vi "Memory.Pointer.In Range.vi"(8 "error in (no error)":errorcluster, 9 "offset":u64 format="%d bytes", 10 "length":i64 format="%d bytes", 11 "Pointer in":refnum<class "Memory.Pointer.lvclass">) -> (0 "error out":errorcluster, 2 "in range?":bool, 3 "Pointer out":refnum<class "Memory.Pointer.lvclass">)   [LabVIEW 2016, in "LabVIEW Memory Manager.lvlib" / "Memory.Pointer.lvclass"]
uses:
  Memory.Pointer.lvclass
  Memory.Pointer.lvclass/Memory.Pointer.ctl
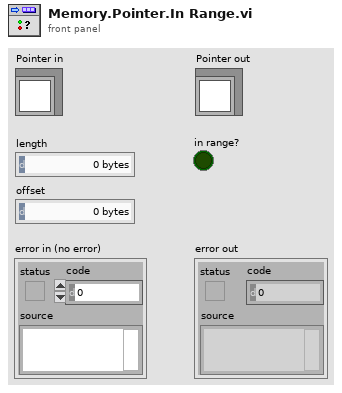
[diagram p1: front panel]
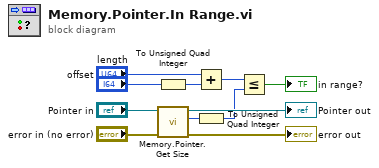
[diagram p0: block diagram]
diagram:
  n1 = To Unsigned Quad Integer(1:"length") -> (0:w6:u64)
  n2 = call "Memory.Pointer.Get Size.vi"("error in (no error)"="error in (no error)", "Pointer in"="Pointer in") -> ("error out"=→"error out":errorcluster, "size"=w7:i64, "Pointer out"=→"Pointer out":refnum<class "Memory.Pointer.lvclass">)  [unwired: 7 in]
  n3 = Add(x="offset", y=w6) -> (x+y=w4:u64)
  n4 = To Unsigned Quad Integer(1:w7) -> (0:w2:u64)
  n5 = Less Or Equal?(x=w4, y=w2) -> (x <= y?=→"in range?":bool)
